vi "stepcontroller.vi"() -> ()   [LabVIEW 2017]
panel:
  out "Boolean 4":bool
  out "Boolean 3":bool
  out "Boolean 2":bool
  in  "Direction":bool
  out "Boolean":bool
  in  "stop":bool
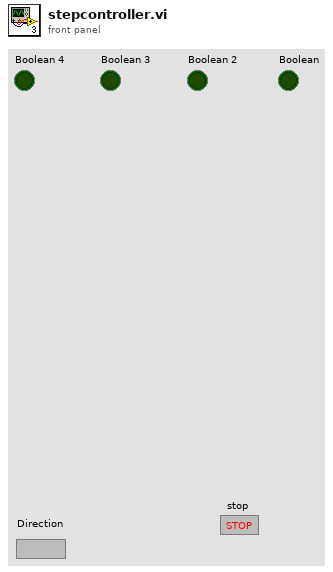
[diagram p1: front panel]
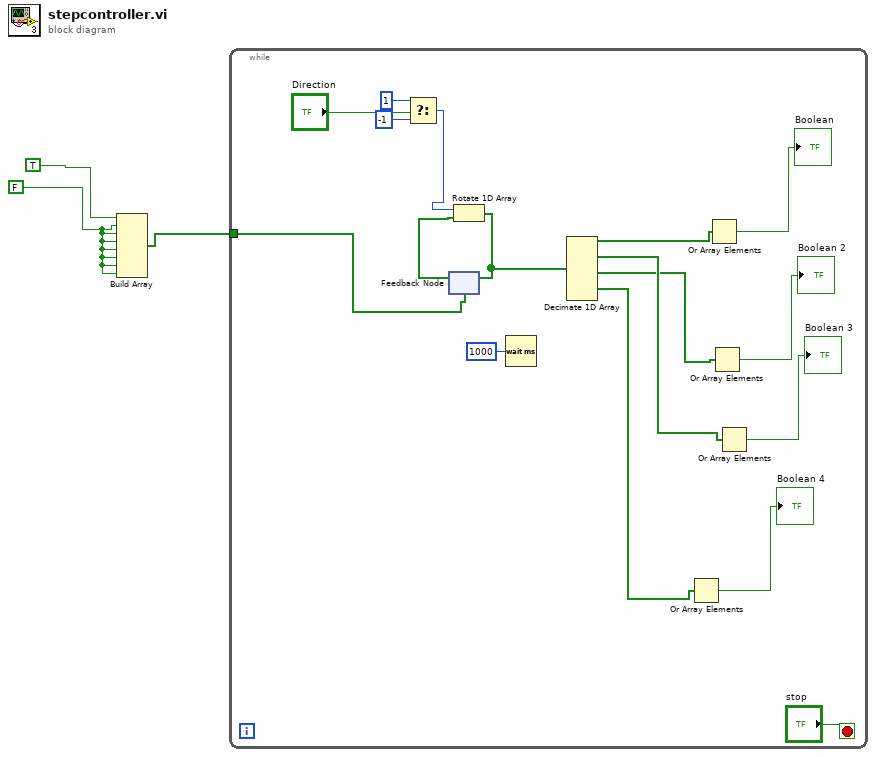
[diagram p0: block diagram]
diagram:
  w1 = FALSE
  n1 = Build Array(TRUE, w1, w1, w1, w1, w1, w1, w1) -> (w3:bool[])
  n2 = while {
    tunnel: w3 -> [w18]
    stop <- "stop" stop-if-true
    n3 = Select(t=1, s="Direction", f=-1) -> (s? t:f=w14:i32)
    n4 = feedback #1(w18) -> (w20:bool[])
    n5 = Rotate 1D Array(1:w20, 2:w14) -> (0:w8:bool[])
    n6 = feedback-in #1(w8) -> ()
    n7 = Wait (ms)(milliseconds to wait=u32 1000) -> ()  [unwired: 1 out]
    n8 = Decimate 1D Array(w8) -> (w7:bool[], w6:bool[], w5:bool[], w4:bool[])  [unwired: 4 out]
    n9 = Or Array Elements(Boolean array=w4) -> (logical OR=→"Boolean 4":bool)
    n10 = Or Array Elements(Boolean array=w7) -> (logical OR=→"Boolean":bool)
    n11 = Or Array Elements(Boolean array=w5) -> (logical OR=→"Boolean 2":bool)
    n12 = Or Array Elements(Boolean array=w6) -> (logical OR=→"Boolean 3":bool)
  }
